vi "CLSUIP_Read Original VI.vi"(1 "VIRetooler.lvclass in":refnum<class "VIRetooler.lvclass">) -> (0 "Original VI":refnum<vi>)   [LabVIEW 2021, in "MemberVICreation.lvlib" / "VIRetooler.lvclass"]
uses:
  <resource>/Framework/Providers/LVClassLibrary/NewAccessors/VIRetooler/VIRetooler.lvclass
  <resource>/Framework/Providers/LVClassLibrary/NewAccessors/VIRetooler/VIRetooler.lvclass/VIRetooler.ctl
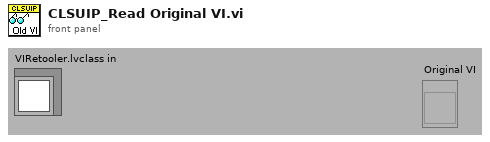
[diagram p1: front panel]
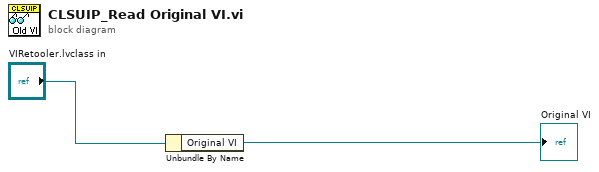
[diagram p0: block diagram]
diagram:
  n1 = Unbundle By Name("VIRetooler.lvclass in") -> ("Original VI"=→"Original VI":refnum<vi>)
